vi "Reinterpret to U16.vi"(8 "error in (no error)":errorcluster, 11 "Array in":u8[](array[numeric])) -> (0 "error out":errorcluster, 3 "Array out":u16[](array[numeric]))   [LabVIEW 2019, in "Picam.lvclass"]
uses:
  Picam.lvclass
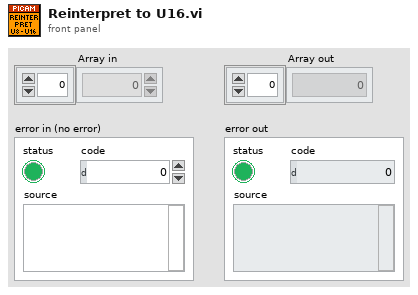
[diagram p1: front panel]
types:
  T1 = enum16{"big-endian, network order", "native, host order", "little-endian"}
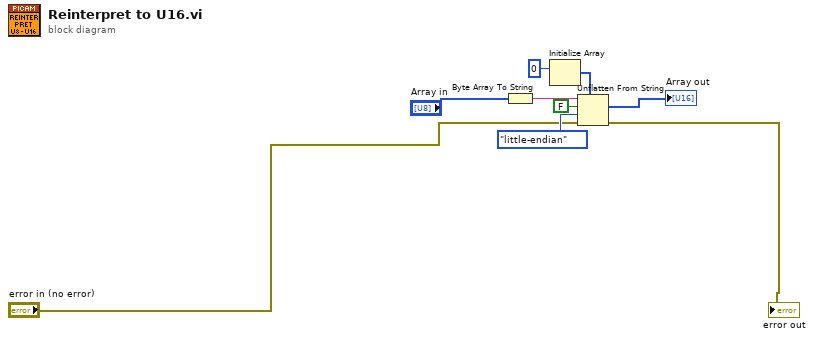
[diagram p0: block diagram]
diagram:
  n1 = Byte Array To String(unsigned byte array="Array in") -> (string=w2:string)
  n2 = Initialize Array(u16 0 ("element")) -> (w3:u16[])  [unwired: 1 in]
  n3 = Unflatten From String(type=w3, binary string=w2, data includes array or string size? (T)=FALSE, byte order (0:big-endian, network order)=T1."little-endian", error in (no error)="error in (no error)") -> (value=→"Array out":u16[], error out=→"error out":errorcluster)  [unwired: 1 out]
